vi "Create Logs Queue.vi"(8 "Error In":errorcluster, 11 "EventLog in":refnum<class "LogsAbstract.lvclass">) -> (0 "Error Out":errorcluster, 3 "EventLog out":refnum<class "LogsAbstract.lvclass">)   [LabVIEW 2019, in "LogsAbstract.lvlib" / "LogsAbstract.lvclass"]
uses:
  LogsAbstract.lvclass
  Classes/EventsAbstract/EventsAbstract.lvclass
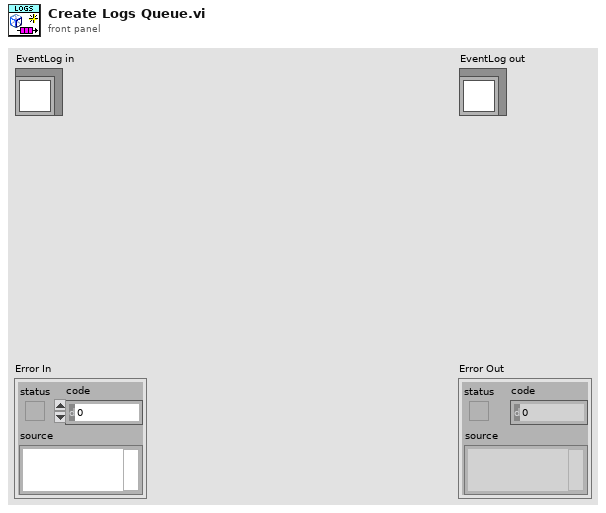
[diagram p1: front panel]
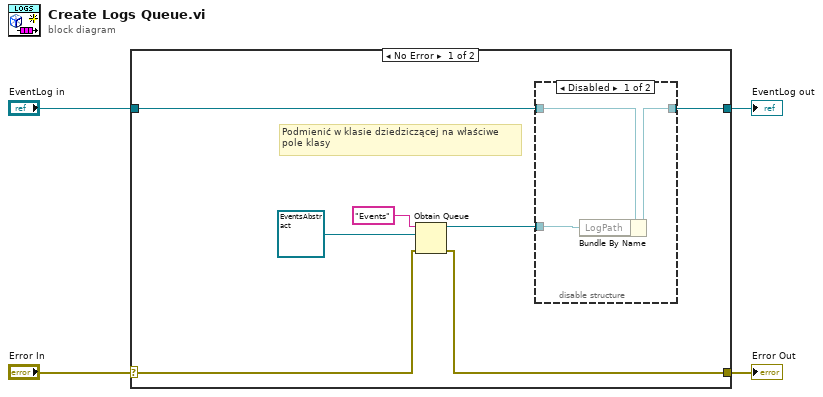
[diagram p0: block diagram]
diagram:
  n1 = case shown="No Error" "Error In" {
    selector: "Error In" -> [w8 w17]
    tunnel: [w7 w17] -> w3
    tunnel: [w6 w16] -> w1
    tunnel: "EventLog in" -> [w11 w16]
    frame No Error {
      # "Podmienić w klasie dziedziczącej na właściwe\npole klasy"
      n2 = Obtain Queue(name (unnamed)="Events", element data type=refnum<class "EventsAbstract.lvclass"> refnum ("Events.lvclass"), error in (no error)=w8) -> (queue out=w5:refnum<queue>, error out=w7:errorcluster)  [unwired: 2 in, 1 out]
      n3 = disable-structure shown="Disabled" {
        disable-tunnel: w11 -> [w14 w15]
        disable-tunnel: [w13 w15] -> w6
        disable-tunnel: w5 -> [w12 _]
        frame Disabled {
          n4 = Bundle By Name(cluster=w14, "LogPath"=w12) -> (w13:refnum<class "LogsAbstract.lvclass">)
        }
        frame Enabled {
        }
      }
    }
    frame Error {
    }
  }
  "Error Out" <- w3
  "EventLog out" <- w1
